vi "TimeTag_LSW_edits_Aug18.vi"() -> ()   [LabVIEW 2015]
doc: "This sample project is built upon the standard state machine template and shows how you could create an application that acquires, analyzes, and presents data. It includes functionality for presenting configuration dialogs, preserving settings between executions, loading and saving data, as well as exporting graph images and text files.\n\nIt is most appropriate for data that is acquired instantly as it does not allow for screen updates mid acquisition nor does it allow for continuous streaming to disk."
uses:
  <vilib>/ptbypt/NI_PtbyPt.lvlib
panel:
  out "real coin cps 10 sec avg":dbl
  out "all coin cps":dbl
  out "real coin cps":dbl
  out "random coin cps":dbl
  out "Real coin cps":dbl(graph)
  out "total coin/sec - total random coin/sec":dbl
  out "total random coincidences/sec":dbl
  out "Total Coin per sec":dbl
  out "Ch2/4 coin/sec":dbl(graph)
  out "Ch2/4 Total Coincidences":dbl
  out "Channel 2 CPS":dbl(graph)
  out "Channel 4 CPS":dbl(graph)
  out "Total Ch2 CPS":dbl
  out "Total Ch4 CPS":dbl
  in  "Averaging":dbl=10.0
  in  "Runs":dbl=100.0
  in  "Pulse TTL 2":bool
  in  "Pulse TTL 1":bool
  in  "Toggle\nTTL 2":bool
  in  "Toggle\nTTL 1":bool
  out "Total Starts":dbl
  in  "Record data":bool
  out "Initial time":dbl
  out "Elapsed time (s)":dbl
  out "FPGA_Run Status":dbl
  out "USB_Open Status":dbl
  out "Channel 4 Total\nCounts":dbl
  out "Channel 3 Total\nCounts":dbl
  out "Channel 2 Total\nCounts":dbl
  out "Channel 1 Total\nCounts":dbl
  in  "File Name":string="C:\\FPGA\\test.txt"
  out "?":dbl
  out "?":dbl
  out "?":dbl
  out "?":dbl
  out "stats":i64[](array[numeric])
  in  "Stop":bool
  out "Channel 4 CPS":dbl(knob) scale=0.0..2000000.0
  out "Channel 3 CPS":dbl(knob) scale=0.0..600.0
  out "Channel 2 CPS":dbl(knob) scale=0.0..700.0
  out "Channel 1 CPS":dbl(knob) scale=0.0..600.0
  # "Starts"
  # "Channel 1"
  # "Channel 2"
  # "Channel 3"
  # "Channel 4"
  # "Coincidence Channels 1 & 2"
  # "Coincidence Channels 1 & 3"
  # "Coincidence Channels 1 & 4"
  # "Coincidence Channels 2 & 3"
  # "Coincidence Channels 2 & 4"
  # "Coincidence Channels 3 & 4"
  # "Coincidence Channels 1 & 2 & 3"
  # "Coincidence Channels 1 & 2 & 4"
  # "Coincidence Channels 1 & 3 & 4"
  # "Coincidence Channels 2 & 3 & 4"
  # "C:\\FPGA_Lauren"
  # "Coincidence Channels 1 & 2 & 3 & 4"
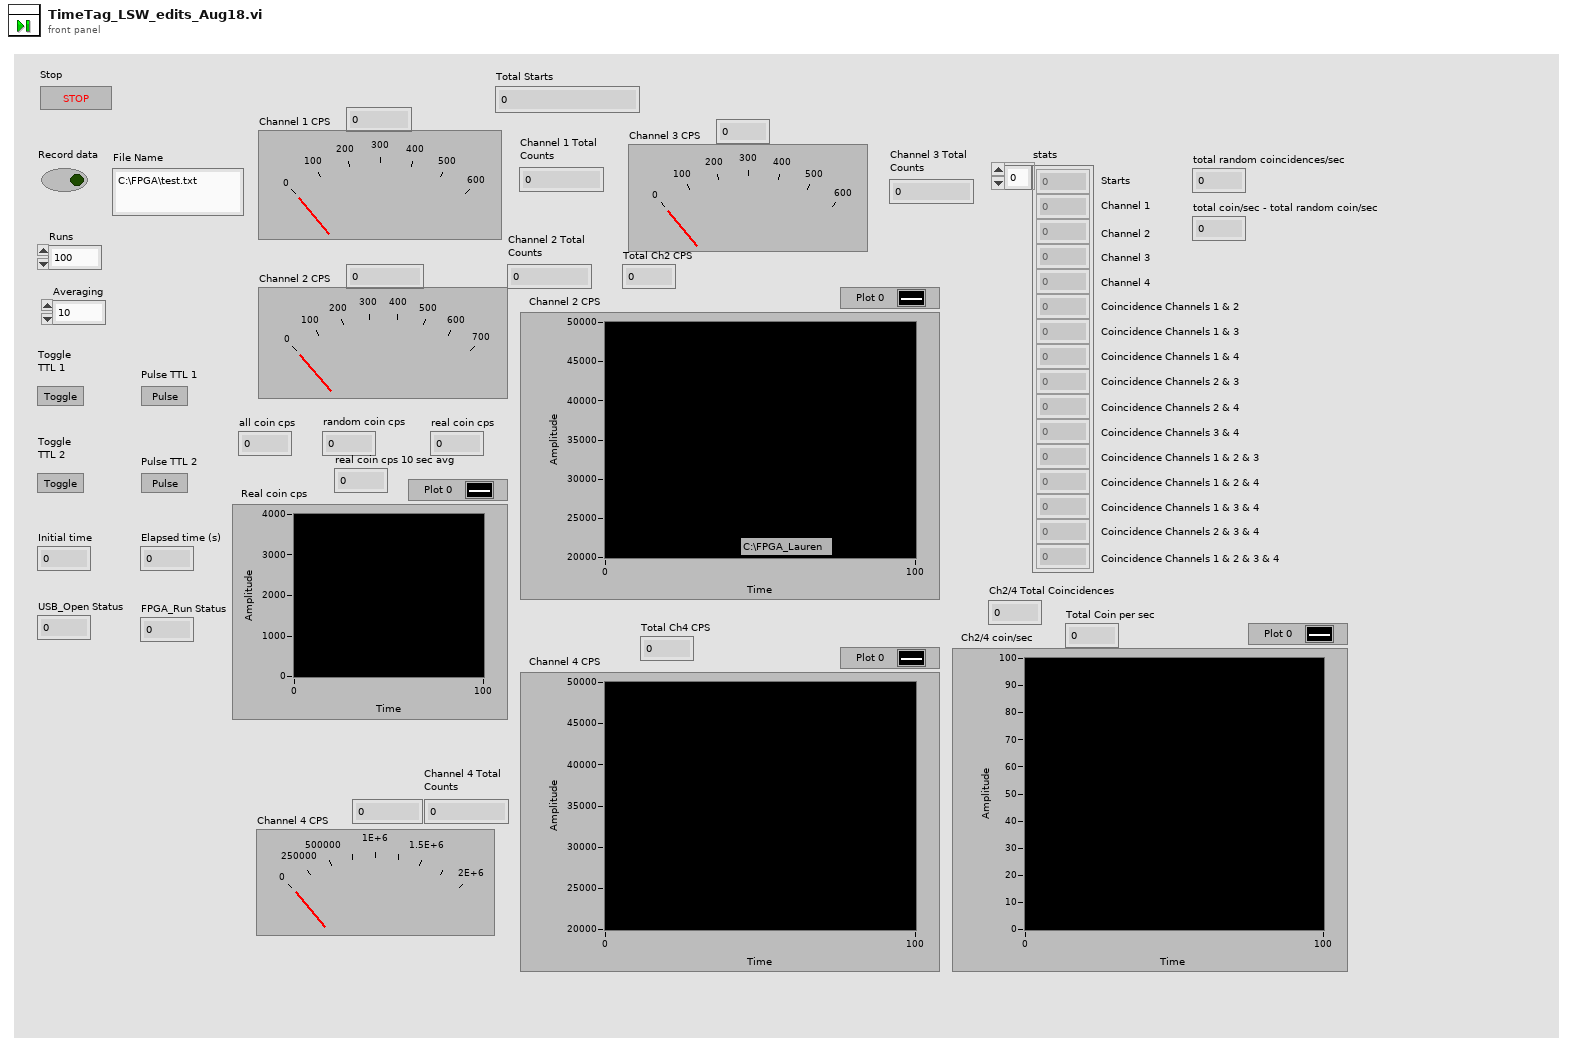
[diagram p1: front panel]
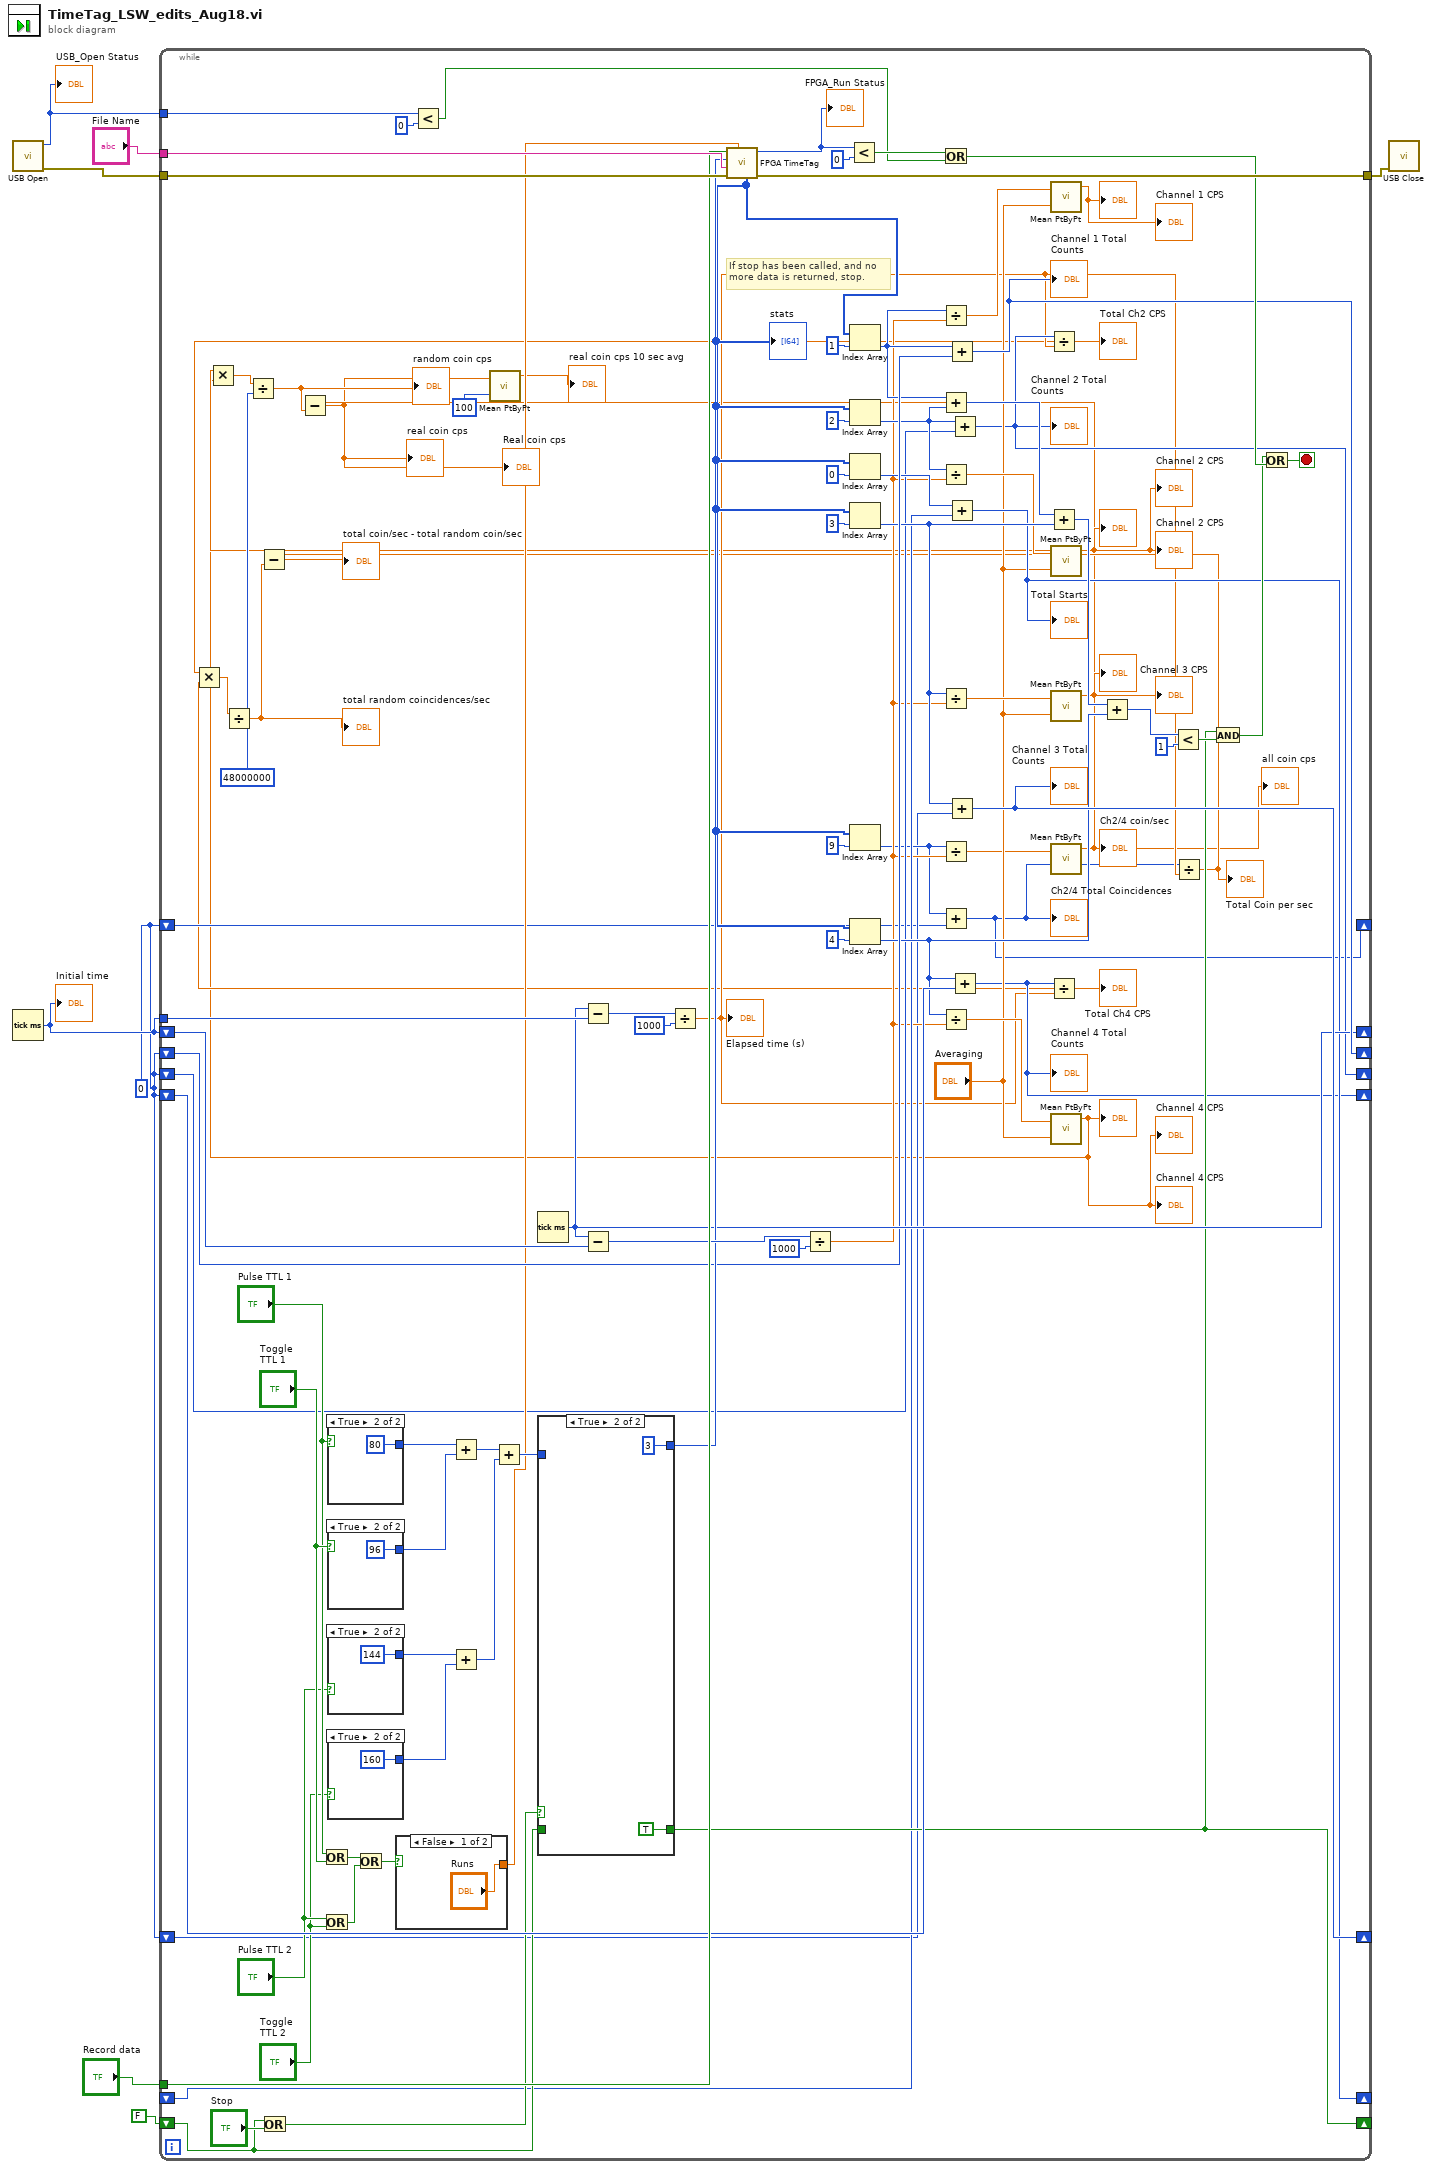
[diagram p0: block diagram]
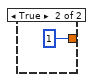
[diagram p2: hidden frame]
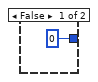
[diagram p3: hidden frame]
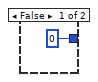
[diagram p4: hidden frame]
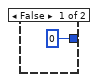
[diagram p5: hidden frame]
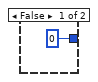
[diagram p6: hidden frame]
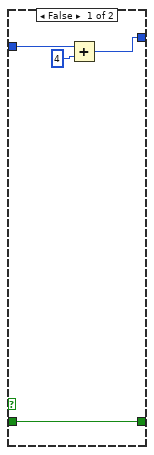
[diagram p7: hidden frame]
diagram:
  w1 = 0
  n1 = call "USB Open.vi"() -> ("error out"=w6:errorcluster, "function return"=w3:i32)  [unwired: 10 in]
  "USB_Open Status" <- w3
  n2 = Tick Count (ms)() -> (millisecond timer value=w4:u32)
  "Initial time" <- w4
  n3 = while {
    tunnel: w4 -> [w103]
    shift-right: [w81] -> _
    shift-left: w1 -> [w77]
    shift-right: [w35] -> _
    shift-left: w1 -> [w31]
    shift-right: [w80] -> _
    shift-left: w1 -> [w27]
    shift-right: [w36] -> _
    shift-left: w1 -> [w76]
    tunnel: w6 -> [w93]
    tunnel: [w94] -> w5
    tunnel: "Record data" -> [w91]
    tunnel: "File Name" -> [w92]
    shift-right: [w78] -> _
    shift-left: w4 -> [w89]
    tunnel: w3 -> [w85]
    shift-right: [w65] -> _
    shift-left: FALSE -> [w62]
    shift-right: [w58] -> _
    shift-left: _ -> [w59]
    shift-right: [w24] -> _
    shift-left: w1 -> [w26]
    stop <- w95 stop-if-true
    w18 = 48000000
    # "If stop has been called, and no\nmore data is returned, stop."
    n4 = Or(x=w62, y="Stop") -> (x .or. y?=w64:bool)
    n5 = Or(x="Pulse TTL 1", y="Toggle\nTTL 1") -> (x .or. y?=w49:bool)
    n6 = Or(x="Pulse TTL 2", y="Toggle\nTTL 2") -> (x .or. y?=w50:bool)
    n7 = case shown="True" "Pulse TTL 1" {
      tunnel: [0 80] -> w57
      frame False {
      }
      frame True {
      }
    }
    n8 = case shown="True" "Toggle\nTTL 1" {
      tunnel: [0 96] -> w56
      frame False {
      }
      frame True {
      }
    }
    n9 = case shown="True" "Pulse TTL 2" {
      tunnel: [0 144] -> w53
      frame False {
      }
      frame True {
      }
    }
    n10 = case shown="True" "Toggle\nTTL 2" {
      tunnel: [0 160] -> w54
      frame False {
      }
      frame True {
      }
    }
    n11 = Or(x=w49, y=w50) -> (x .or. y?=w51:bool)
    n12 = case shown="False" w51 {
      tunnel: ["Runs" 1] -> w47
      frame False {
      }
      frame True {
      }
    }
    n13 = Less?(x=w85, y=0) -> (x < y?=w83:bool)
    n14 = Add(x=w57, y=w56) -> (x+y=w55:i32)
    n15 = Add(x=w53, y=w54) -> (x+y=w52:i32)
    n16 = Add(x=w55, y=w52) -> (x+y=w48:i32)
    n17 = Tick Count (ms)() -> (millisecond timer value=w78:u32)
    n18 = case shown="True" w64 {
      tunnel: [w115 3] -> w79
      tunnel: [w117 TRUE] -> w65
      tunnel: w62 -> [w117 _]
      tunnel: w48 -> [w114 _]
      frame False {
        n19 = Add(x=w114, y=4) -> (x+y=w115:i32)
      }
      frame True {
      }
    }
    n20 = Subtract(x=w78, y=w103) -> (x-y=w102:u32)
    n21 = Subtract(x=w78, y=w89) -> (x-y=w88:u32)
    n22 = Divide(x=w102, y=1000) -> (x/y=w25:dbl)
    "Elapsed time (s)" <- w25
    n23 = call "FPGA TimeTag.vi"("runs"=w47, "error in (no error)"=w93, "fileName"=w92, "fpgaCommand"=w79, "saveData"=w91) -> ("error out"=w94:errorcluster, "function return"=w90:i32, "stats"=w33:i64[])  [unwired: 4 in]
    "stats" <- w33
    "FPGA_Run Status" <- w90
    n24 = Divide(x=w88, y=1000) -> (x/y=w30:dbl)
    n25 = Less?(x=w90, y=0) -> (x < y?=w84:bool)
    n26 = Index Array(array=w33, index=1) -> (element=w68:i64)
    n27 = Index Array(array=w33, index=2) -> (element=w75:i64)
    n28 = Index Array(array=w33, index=0) -> (element=w60:i64)
    n29 = Index Array(array=w33, index=3) -> (element=w71:i64)
    n30 = Index Array(array=w33, index=9) -> (element=w28:i64)
    n31 = Index Array(array=w33, index=4) -> (element=w72:i64)
    n32 = Or(x=w84, y=w83) -> (x .or. y?=w82:bool)
    n33 = Divide(x=w68, y=w30) -> (x/y=w42:dbl)
    n34 = Add(x=w68, y=w75) -> (x+y=w70:i64)
    n35 = Divide(x=w75, y=w30) -> (x/y=w41:dbl)
    n36 = Divide(x=w71, y=w30) -> (x/y=w40:dbl)
    n37 = Divide(x=w28, y=w30) -> (x/y=w29:dbl)
    n38 = Add(x=w28, y=w26) -> (x+y=w24:i64)
    "Ch2/4 Total Coincidences" <- w24
    n39 = Divide(x=w72, y=w30) -> (x/y=w38:dbl)
    n40 = Add(x=w68, y=w77) -> (x+y=w81:i64)
    "Channel 1 Total\nCounts" <- w81
    n41 = Add(x=w60, y=w59) -> (x+y=w58:i64)
    "Total Starts" <- w58
    n42 = Add(x=w71, y=w27) -> (x+y=w80:i64)
    "Channel 3 Total\nCounts" <- w80
    n43 = Add(x=w75, y=w31) -> (x+y=w35:i64)
    "Channel 2 Total\nCounts" <- w35
    n44 = Add(x=w72, y=w76) -> (x+y=w36:i64)
    "Channel 4 Total\nCounts" <- w36
    n45 = Divide(x=w35, y=w25) -> (x/y=w21:dbl)
    "Total Ch2 CPS" <- w21
    n46 = Add(x=w70, y=w71) -> (x+y=w74:i64)
    n47 = Divide(x=w36, y=w25) -> (x/y=w20:dbl)
    "Total Ch4 CPS" <- w20
    n48 = Multiply(x=w21, y=w20) -> (x*y=w19:dbl)
    n49 = Divide(x=w19, y=w18) -> (x/y=w22:dbl)
    "total random coincidences/sec" <- w22
    n50 = call <vilib>:"Mean PtByPt.vi"("x"=w42, "sample length"="Averaging") -> ("mean"=→"Channel 1 CPS" →"?":dbl)  [unwired: 2 in, 1 out]
    n51 = call <vilib>:"Mean PtByPt.vi"("x"=w41, "sample length"="Averaging") -> ("mean"=w17:dbl)  [unwired: 2 in, 1 out]
    "Channel 2 CPS" <- w17
    "?" <- w17
    "Channel 2 CPS" <- w17
    n52 = call <vilib>:"Mean PtByPt.vi"("x"=w40, "sample length"="Averaging") -> ("mean"=→"Channel 3 CPS" →"?":dbl)  [unwired: 2 in, 1 out]
    n53 = call <vilib>:"Mean PtByPt.vi"("x"=w29) -> ("mean"=w12:dbl)  [unwired: 3 in, 1 out]
    "Ch2/4 coin/sec" <- w12
    "all coin cps" <- w12
    n54 = call <vilib>:"Mean PtByPt.vi"("x"=w38, "sample length"="Averaging") -> ("mean"=w16:dbl)  [unwired: 2 in, 1 out]
    "Channel 4 CPS" <- w16
    "?" <- w16
    "Channel 4 CPS" <- w16
    n55 = Multiply(x=w17, y=w16) -> (x*y=w15:dbl)
    n56 = Divide(x=w15, y=w18) -> (x/y=w14:dbl)
    "random coin cps" <- w14
    n57 = Subtract(x=w12, y=w14) -> (x-y=w11:dbl)
    "Real coin cps" <- w11
    "real coin cps" <- w11
    n58 = call <vilib>:"Mean PtByPt.vi"("x"=w11, "sample length"=100) -> ("mean"=→"real coin cps 10 sec avg":dbl)  [unwired: 2 in, 1 out]
    n59 = Add(x=w74, y=w72) -> (x+y=w73:i64)
    n60 = Less?(x=w73, y=1) -> (x < y?=w67:bool)
    n61 = Divide(x=w24, y=w25) -> (x/y=w23:dbl)
    "Total Coin per sec" <- w23
    n62 = Subtract(x=w23, y=w22) -> (x-y=→"total coin/sec - total random coin/sec":dbl)
    n63 = And(x=w65, y=w67) -> (x .and. y?=w66:bool)
    n64 = Or(x=w66, y=w82) -> (x .or. y?=w95:bool)
  }
  n65 = call "USB Close.vi"("error in (no error)"=w5) -> ()  [unwired: 9 in, 2 out]
